vi "DMM_test.vi"() -> ()   [LabVIEW 2020]
uses:
  <instrlib>/niDMM/nidmm.llb/niDMM Resolution in Digits.ctl
  <instrlib>/niDMM/nidmm.llb/niDMM Function.ctl
  <instrlib>/niDMM/nidmm.llb/niDMM Configure Measurement Digits.vi
panel:
  out "error out":errorcluster
  out "Measurement (Volts)":dbl format="%_7p"
  in  "Range (Volts)":dbl=10.0 format="%.2p"
  in  "Device Name":refnum<k15>="NI_DMM"
  out "Signal Out of Range":bool
  in  "Measurement Type":T1
  in  "Resolution in Digits":T2=5.5 items=["3 1/2"=3.5, "4 1/2"=4.5, "5 1/2"=5.5, "6 1/2"=6.5, "7 1/2"=7.5]
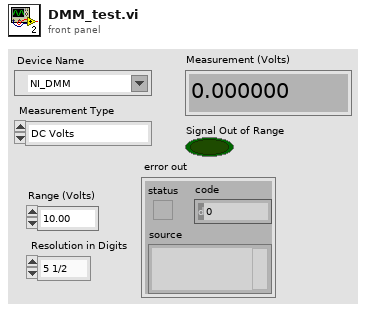
[diagram p1: front panel]
types:
  T1 = typedef "niDMM Function.ctl" = enum16{"DC Volts", "AC Volts", "DC Current", "AC Current", "2-wire Resistance", "4-wire Resistance", "Diode", "Frequency", "Period", "AC Volts DC Coupled", "Capacitance", "Inductance", "Temperature"}
  T2 = typedef "niDMM Resolution in Digits.ctl" = dbl
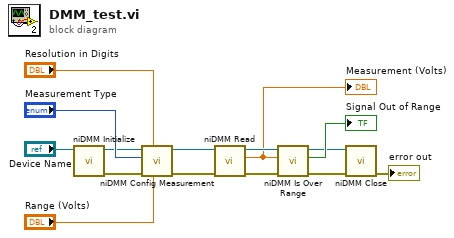
[diagram p0: block diagram]
diagram:
  n1 = call <instrlib>:"niDMM Initialize.vi"("Instrument Descriptor"="Device Name") -> ("error out"=w3:errorcluster, "instrument handle out"=w2:refnum<k15>)  [unwired: 9 in]
  n2 = call-poly <instrlib>:"niDMM Config Measurement.vi"("Range"="Range (Volts)", "Resolution in Digits"="Resolution in Digits", "error in (no error)"=w3, "Function"="Measurement Type", "instrument handle"=w2) -> ("error out"=w10:errorcluster, "instrument handle out"=w11:refnum<k15>)  [unwired: 5 in]
  n3 = call <instrlib>:"niDMM Read.vi"("error in (no error)"=w10, "instrument handle"=w11) -> ("error out"=w9:errorcluster, "Measurement"=w7:dbl, "instrument handle out"=w8:refnum<k15>)  [unwired: 7 in]
  "Measurement (Volts)" <- w7
  n4 = call <instrlib>:"niDMM Is Over Range.vi"("error in (no error)"=w9, "Measurement"=w7, "instrument handle"=w8) -> ("error out"=w13:errorcluster, "Over Range?"=→"Signal Out of Range":bool, "instrument handle out"=w12:refnum<k15>)  [unwired: 6 in]
  n5 = call <instrlib>:"niDMM Close.vi"("error in (no error)"=w13, "instrument handle"=w12) -> ("error out"=→"error out":errorcluster)  [unwired: 9 in]
